vi "Lookup by ID.vi"(8 "error in (no error)":errorcluster, 10 "ID":i64, 11 "Challenge DB in":refnum<class "Challenge DB.lvclass">) -> (0 "error out":errorcluster, 1 "Found?":bool, 2 "Challenge":refnum<class "Challenge.lvclass">, 3 "Challenge DB out":refnum<class "Challenge DB.lvclass">)   [LabVIEW 2020, in "Summer of LabVIEW.lvlib" / "Challenge DB.lvclass"]
uses:
  Challenge DB.lvclass
  Challenge DB.lvclass/Challenge DB.ctl
  Challenge/Challenge.lvclass
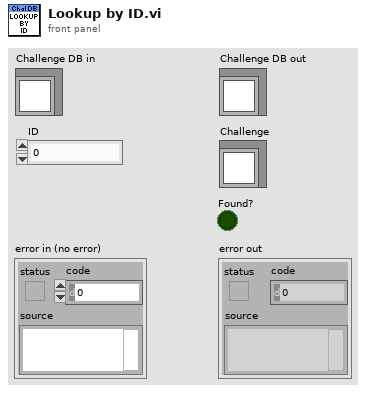
[diagram p1: front panel]
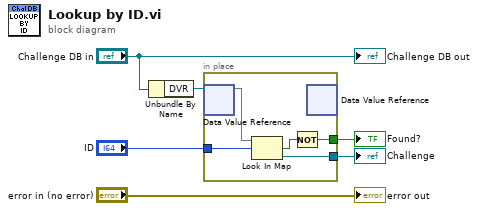
[diagram p0: block diagram]
diagram:
  n1 = Unbundle By Name("Challenge DB in") -> ("DVR"=w5:refnum<data-value>)
  n2 = in-place {
    in-place-border: "ID" -> [w10]
    in-place-border: [w9] -> w2
    in-place-border: [w7] -> w1
    n3 = in-place-dvr #1(w5) -> (w11:map{i64, refnum<class "Challenge.lvclass">})  [unwired: 1 out]
    n4 = Look In Map(map=w11, key=w10) -> (key not found?=w8:bool, value=w9:refnum<class "Challenge.lvclass">)  [unwired: 1 in]
    n5 = Not(x=w8) -> (.not. x?=w7:bool)
    n6 = in-place-dvr #1() -> ()  [unwired: 1 in, 2 out]
  }
  "Challenge" <- w2
  "Found?" <- w1
  "error out" <- "error in (no error)"
  "Challenge DB out" <- "Challenge DB in"
